vi "Do.vi"(8 "error in (no error)":errorcluster, 10 "Actor in":refnum<class "Actor.lvclass">, 11 "Create Ref Message":refnum<class "Create Ref Message.lvclass">) -> (0 "error out":errorcluster, 2 "Actor out":refnum<class "Actor.lvclass">)   [LabVIEW 2019, in "Create Ref Message.lvclass"]
doc: "(<B>Filename</B>: Actor Framework.lvlib:Message.lvclass:Do.vi)\n\nDefines what a message does when it is received by an actor. Generally, a message instructs an actor to invoke one of its methods. By default, this method does nothing. A child class must override it to define behavior. Create a child class by using the Actor Framework Message Maker dialog box."
uses:
  <vilib>/gpm_packages/@cs/Network-interface/Source/Create Ref Message/Create Ref Message.lvclass
  <vilib>/ActorFramework/Actor/Actor.lvclass
  <vilib>/gpm_packages/@cs/Network-interface/Source/Create Ref Message/Create Ref Message.lvclass/Create Ref Message.ctl
  <vilib>/gpm_packages/@cs/Network-interface/Source/Connection Factory Session/ConnectionFactorySession/ConnectionFactorySession.lvclass
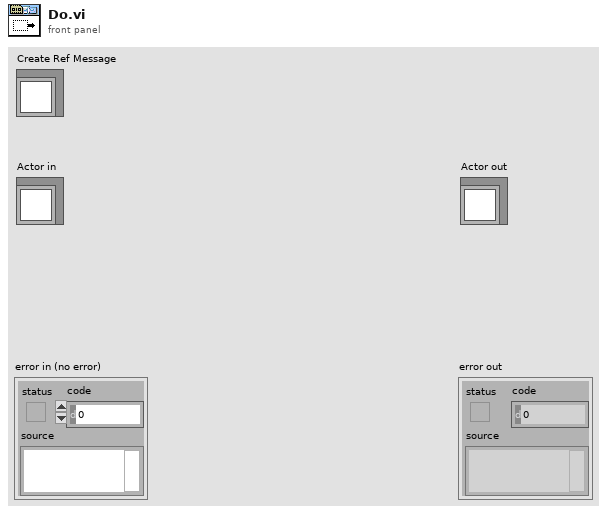
[diagram p1: front panel]
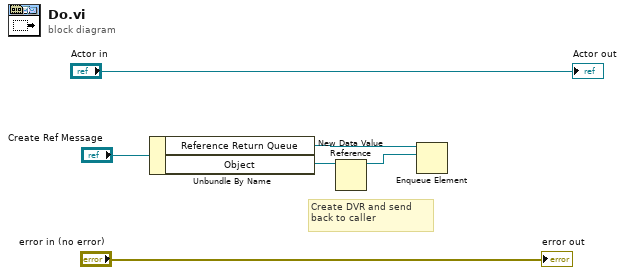
[diagram p0: block diagram]
diagram:
  # "Create DVR and send back to caller"
  n1 = Unbundle By Name("Create Ref Message") -> ("Reference Return Queue"=w3:refnum<queue>, "Object"=w1:refnum<class>)
  n2 = New Data Value Reference(data value=w1) -> (data value reference=w2:refnum<data-value>)  [unwired: 1 in, 1 out]
  n3 = Enqueue Element(queue=w3, element=w2) -> ()  [unwired: 2 in, 3 out]
  "error out" <- "error in (no error)"
  "Actor out" <- "Actor in"
